vi "set seq channel writer or reader.vi"(7 "module GUID":string, 8 "error in":errorcluster, 9 "channel":refnum<class "TBM channel.lvclass">, 10 "tag descriptor":refnum<class "tag descriptor.lvclass">, 11 "sequencer config in":refnum<class "base TBM sequencer configuration.lvclass">) -> (0 "error out":errorcluster, 3 "sequencer config out":refnum<class "base TBM sequencer configuration.lvclass">)   [LabVIEW 2014, in "base TBM sequencer configuration.lvclass"]
uses:
  base TBM sequencer configuration.lvclass
  <vilib>/NI/Tag Bus Module Framework/channel/TBM channel.lvclass
  <vilib>/NI/Configuration Framework/NISE_CEF_TreeControl.lvlib
  <vilib>/NI/Tag Bus/tag/tag descriptor.lvclass
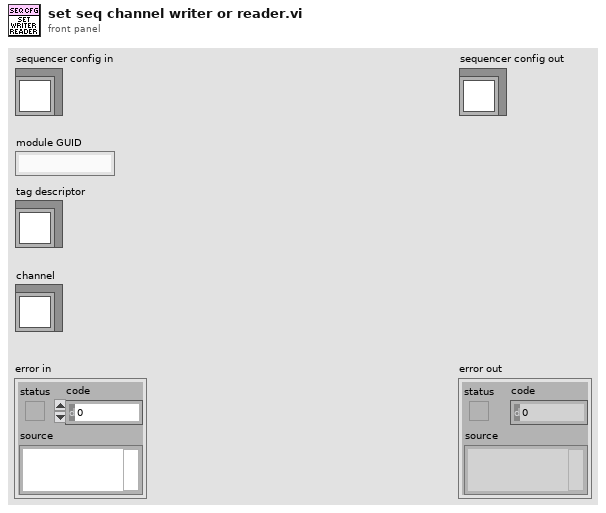
[diagram p1: front panel]
types:
  T1 = typedef "base TBM sequencer configuration.lvclass/Tag Info.ctl" = cluster{"Channel":refnum<class "TBM channel.lvclass">, "Writers":string[], "Readers":string[], "Owning ID":string}
  T2 = typedef "TBM channel.lvclass/channel classification.ctl" = enum16{"input data", "output data", "processing parameter", "processing result"}
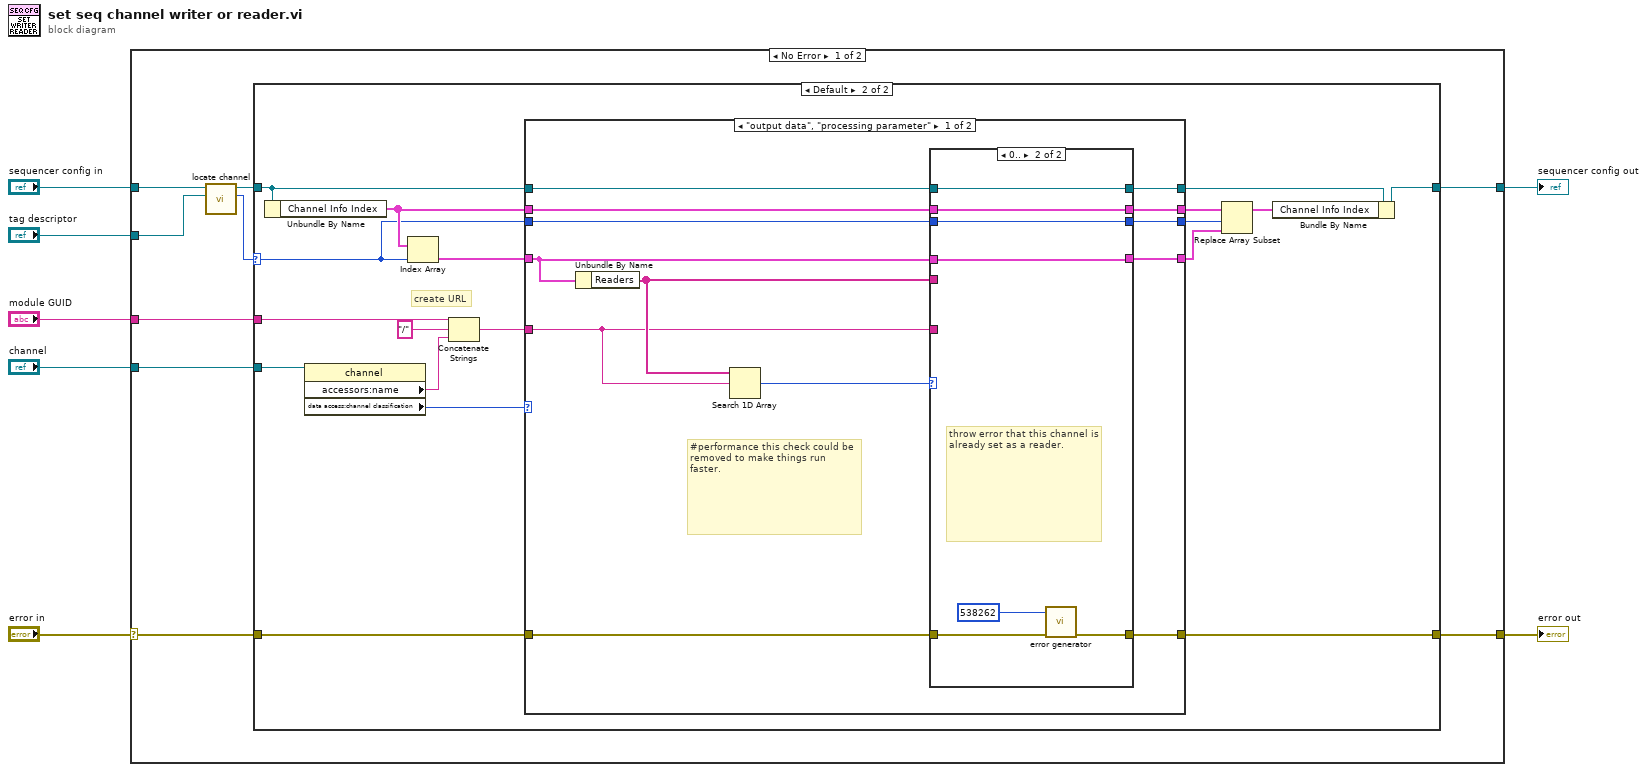
[diagram p0: block diagram]
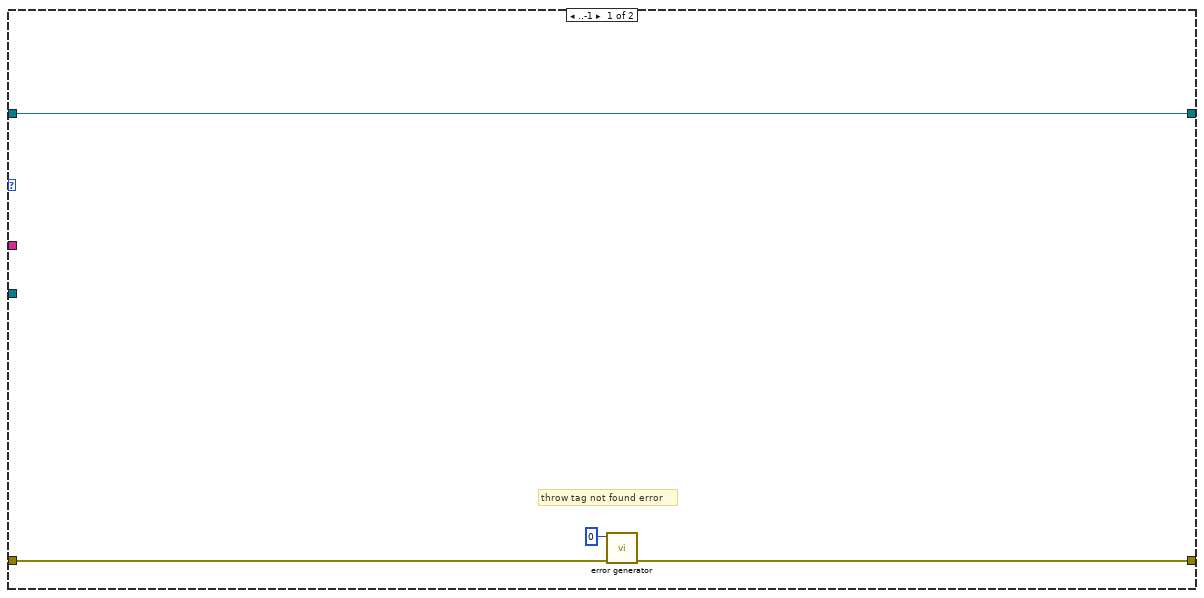
[diagram p2: hidden frame]
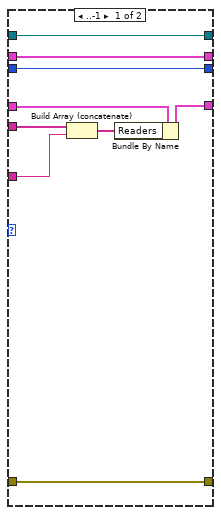
[diagram p3: hidden frame]
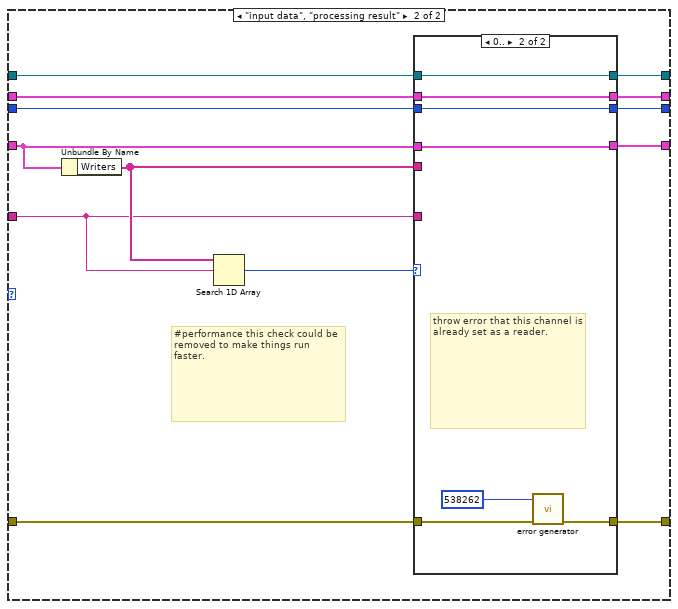
[diagram p4: hidden frame]
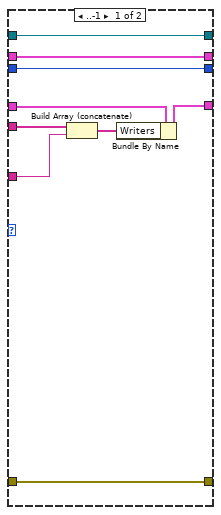
[diagram p5: hidden frame]
diagram:
  n1 = case shown="No Error" "error in" {
    selector: "error in" -> [w11 w98]
    tunnel: [w9 w98] -> w6
    tunnel: [w8 w97] -> w4
    tunnel: "sequencer config in" -> [w16 w97]
    tunnel: "tag descriptor" -> [w15 _]
    tunnel: "module GUID" -> [w12 _]
    tunnel: "channel" -> [w13 _]
    frame No Error {
      n2 = call "locate channel.vi"("tag descriptor"=w15, "sequencer config in"=w16) -> ("index"=w10:i32, "sequencer config out"=w14:refnum<class "base TBM sequencer configuration.lvclass">)  [unwired: 8 in]
      n3 = case shown="Default" w10 {
        selector: w10 -> [_ w29]
        tunnel: w14 -> [w20 w28]
        tunnel: w13 -> [_ w38]
        tunnel: w12 -> [_ w36]
        tunnel: w11 -> [w19 w31]
        tunnel: [w18 w27] -> w9
        tunnel: [w20 w21] -> w8
        frame ..-1 {
          # "throw tag not found error"
          n4 = call <vilib>:"error generator.vi"("error in"=w19, "error code (0)"=0) -> ("error out"=w18:errorcluster)  [unwired: 7 in]
        }
        frame Default {
          # "create URL"
          n5 = Unbundle By Name(w28) -> ("Channel Info Index"=w30:T1[])
          n6 = property class="channel"(reference=w38) -> ("accessors:name"=w35:string, "data access:channel classification"=w34:T2)  [unwired: 1 in, 2 out]
          n7 = Index Array(array=w30, index=w29) -> (element=w32:T1)
          n8 = Concatenate Strings(w36, "/" ("string"), w35) -> (w33:string)
          n9 = case shown="\"output data\", \"processing parameter\"" w34 {
            tunnel: w33 -> [w40 w69]
            tunnel: w32 -> [w51 w80]
            tunnel: w31 -> [w47 w76]
            tunnel: w30 -> [w44 w73]
            tunnel: w29 -> [w42 w71]
            tunnel: w28 -> [w50 w79]
            tunnel: [w49 w78] -> w23
            tunnel: [w48 w77] -> w24
            tunnel: [w46 w75] -> w27
            tunnel: [w45 w74] -> w25
            tunnel: [w43 w72] -> w26
            frame "output data", "processing parameter" {
              # "#performance this check could be removed to make things run faster."
              n10 = Unbundle By Name(w51) -> ("Readers"=w41:string[])
              n11 = Search 1D Array(1D array=w41, element=w40) -> (index of element=w39:i32)  [unwired: 1 in]
              n12 = case shown="0.." w39 {
                tunnel: w41 -> [w60 _]
                tunnel: w40 -> [w59 _]
                tunnel: w51 -> [w58 w66]
                tunnel: w50 -> [w56 w67]
                tunnel: [w56 w67] -> w49
                tunnel: [w55 w66] -> w48
                tunnel: w47 -> [w54 w63]
                tunnel: [w54 w62] -> w46
                tunnel: [w53 w65] -> w45
                tunnel: w44 -> [w53 w65]
                tunnel: [w52 w64] -> w43
                tunnel: w42 -> [w52 w64]
                frame ..-1 {
                  n13 = Build Array (concatenate)(w60, w59) -> (w57:string[])
                  n14 = Bundle By Name(cluster=w58, "Readers"=w57) -> (w55:T1)
                }
                frame 0.. {
                  # "throw error that this channel is already set as a reader."
                  n15 = call <vilib>:"error generator.vi"("error in"=w63, "error code (0)"=538262) -> ("error out"=w62:errorcluster)  [unwired: 7 in]
                }
              }
            }
            frame "input data", "processing result" {
              # "#performance this check could be removed to make things run faster."
              n16 = Unbundle By Name(w80) -> ("Writers"=w70:string[])
              n17 = Search 1D Array(1D array=w70, element=w69) -> (index of element=w68:i32)  [unwired: 1 in]
              n18 = case shown="0.." w68 {
                tunnel: w70 -> [w89 _]
                tunnel: w69 -> [w88 _]
                tunnel: w80 -> [w87 w95]
                tunnel: w79 -> [w85 w96]
                tunnel: [w85 w96] -> w78
                tunnel: [w84 w95] -> w77
                tunnel: w76 -> [w83 w92]
                tunnel: [w83 w91] -> w75
                tunnel: [w82 w94] -> w74
                tunnel: w73 -> [w82 w94]
                tunnel: [w81 w93] -> w72
                tunnel: w71 -> [w81 w93]
                frame ..-1 {
                  n19 = Build Array (concatenate)(w89, w88) -> (w86:string[])
                  n20 = Bundle By Name(cluster=w87, "Writers"=w86) -> (w84:T1)
                }
                frame 0.. {
                  # "throw error that this channel is already set as a reader."
                  n21 = call <vilib>:"error generator.vi"("error in"=w92, "error code (0)"=538262) -> ("error out"=w91:errorcluster)  [unwired: 7 in]
                }
              }
            }
          }
          n22 = Replace Array Subset(array=w25, new element=w24, index=w26) -> (w22:T1[])
          n23 = Bundle By Name(cluster=w23, "Channel Info Index"=w22) -> (w21:refnum<class "base TBM sequencer configuration.lvclass">)
        }
      }
    }
    frame Error {
    }
  }
  "error out" <- w6
  "sequencer config out" <- w4
